vi "GetGraphTypeInfo.vi"(0 "reference in":refnum<class "UseCaseDiagramGraph.lvclass">, 5 "error in (no error)":errorcluster) -> (14 "reference out":refnum<class "UseCaseDiagramGraph.lvclass">, 15 "GraphTypeName":string, 16 "NodeTypes":refnum<class "AbstractNode.lvclass">[](array[class]), 17 "EdgeTypes":refnum<class "AbstractEdge.lvclass">[](array[class]), 18 "GraphTypeUserName":string, 19 "error out":errorcluster)   [LabVIEW 2020, in "UseCaseDiagramGraph.lvclass"]
uses:
  <resource>/Framework/Providers/Open_GDS/UML/UseCaseDiagramGraph_class/UseCaseDiagramGraph.lvclass
  <resource>/Framework/Providers/Open_GDS/UML/AbstractNode_class/AbstractNode.lvclass
  <resource>/Framework/Providers/Open_GDS/UML/AbstractEdge_class/AbstractEdge.lvclass
  <resource>/Framework/Providers/Open_GDS/UML/NoteNode_class/NoteNode.lvclass
  C:/Program Files (x86)/National Instruments/LabVIEW 2020/resource/Framework/Providers/Open_GDS/UML/AbstractNode_class/AbstractNode.lvclass
  <resource>/Framework/Providers/Open_GDS/UML/NoteEdge_class/NoteEdge.lvclass
  C:/Program Files (x86)/National Instruments/LabVIEW 2020/resource/Framework/Providers/Open_GDS/UML/GeneralPathEdge_class/GeneralPathEdge.lvclass
  <resource>/Framework/Providers/Open_GDS/UML/SystemNode_class/SystemNode.lvclass
  <resource>/Framework/Providers/Open_GDS/UML/ActorNode_class/ActorNode.lvclass
  <resource>/Framework/Providers/Open_GDS/UML/UseCaseNode_class/UseCaseNode.lvclass
  <resource>/Framework/Providers/Open_GDS/UML/SegmentedLineEdge_class/SegmentedLineEdge.lvclass
  <resource>/Framework/Providers/Open_GDS/UML/PointNode_class/PointNode.lvclass
  <resource>/Framework/Providers/Open_GDS/UML/GeneralPathEdge_class/GeneralPathEdge.lvclass
  C:/Program Files (x86)/National Instruments/LabVIEW 2020/resource/Framework/Providers/Open_GDS/UML/AbstractEdge_class/AbstractEdge.lvclass
  <resource>/Framework/Providers/Open_GDS/UML/Graph_class/Graph.lvclass
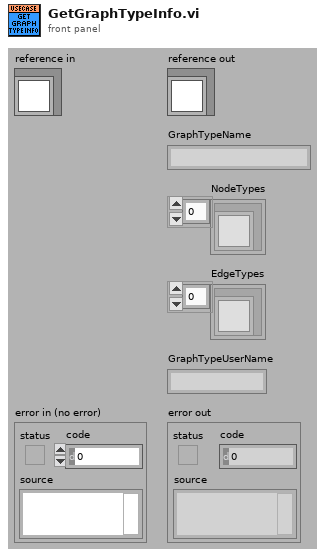
[diagram p1: front panel]
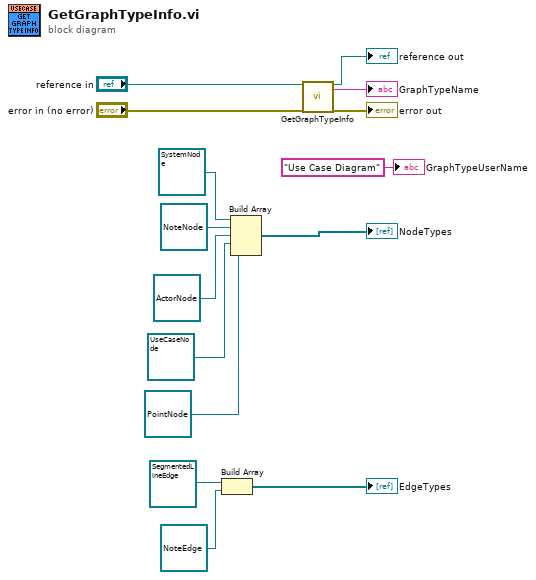
[diagram p0: block diagram]
diagram:
  n1 = Build Array(refnum<class "SegmentedLineEdge.lvclass"> refnum ("SegmentedLineEdge.lvclass"), refnum<class "NoteEdge.lvclass"> refnum ("NoteEdge.lvclass")) -> (→"EdgeTypes":refnum<class "GeneralPathEdge.lvclass">[])
  n2 = Build Array(refnum<class "SystemNode.lvclass"> refnum ("SystemNode.lvclass"), refnum<class "NoteNode.lvclass"> refnum ("NoteNode.lvclass"), refnum<class "ActorNode.lvclass"> refnum ("ActorNode.lvclass"), refnum<class "UseCaseNode.lvclass"> refnum ("UseCaseNode.lvclass"), refnum<class "PointNode.lvclass"> refnum ("PointNode.lvclass")) -> (→"NodeTypes":refnum<class "AbstractNode.lvclass">[])
  n3 = call-parent "GetGraphTypeInfo.vi"("reference in"="reference in", "error in (no error)"="error in (no error)") -> ("reference out"=→"reference out":refnum<class "UseCaseDiagramGraph.lvclass">, "GraphTypeName"=→"GraphTypeName":string, "error out"=→"error out":errorcluster)  [unwired: 12 in, 3 out]
  "GraphTypeUserName" <- "Use Case Diagram" ("GraphTypeUserName")
